vi "FileAppenderConfigDTOFromNative.vi"(8 "error in (no error)":errorcluster, 11 "FileAppenderConfig":T1={"common"={"id"="", "threshold"=enum."INFO", "filter"={"mode"=enum."Mirror", "levelMin"=enum."INFO", "levelMax"=enum."INFO", "tagPrefix"=""}, "queueBound"=0, "dropPolicy"=enum."DropOldest", "useUTC"=FALSE}, "file"={"rootFolder"=path "", "maxFileSize"=0, "maxFileCount"=0, "baseName"="", "extension"="", "delimiter"="", "calendarFolderTree"=FALSE}}) -> (0 "error out":errorcluster, 3 "FileAppenderConfigDTO":T8={"common"={"id"="", "threshold"="INFO", "filter"={"mode"="Mirror", "levelMin"="INFO", "levelMax"="INFO", "tagPrefix"=""}, "queueBound"=0, "dropPolicy"="DropOldest", "useUTC"=FALSE}, "file"={"rootFolder"="", "maxFileSize"=0, "maxFileCount"=0, "baseName"="", "extension"="", "delimiter"="", "calendarFolderTree"=FALSE}})   [LabVIEW 2026, in "Lumberjack.lvlib"]
uses:
  Lumberjack.lvlib
  TypeDefs/ConfigDTO/FilterDTO.ctl
  TypeDefs/ConfigDTO/AppenderConfigDTO.ctl
  TypeDefs/ConfigDTO/FileAppenderConfigDTO.ctl
  TypeDefs/ConfigDTO/FileConfigDTO.ctl
  TypeDefs/Severity.ctl
  TypeDefs/FilterMode.ctl
  TypeDefs/Filter.ctl
  TypeDefs/DropPolicy.ctl
  TypeDefs/AppenderConfig.ctl
  TypeDefs/FileAppenderConfig.ctl
  TypeDefs/FileConfig.ctl
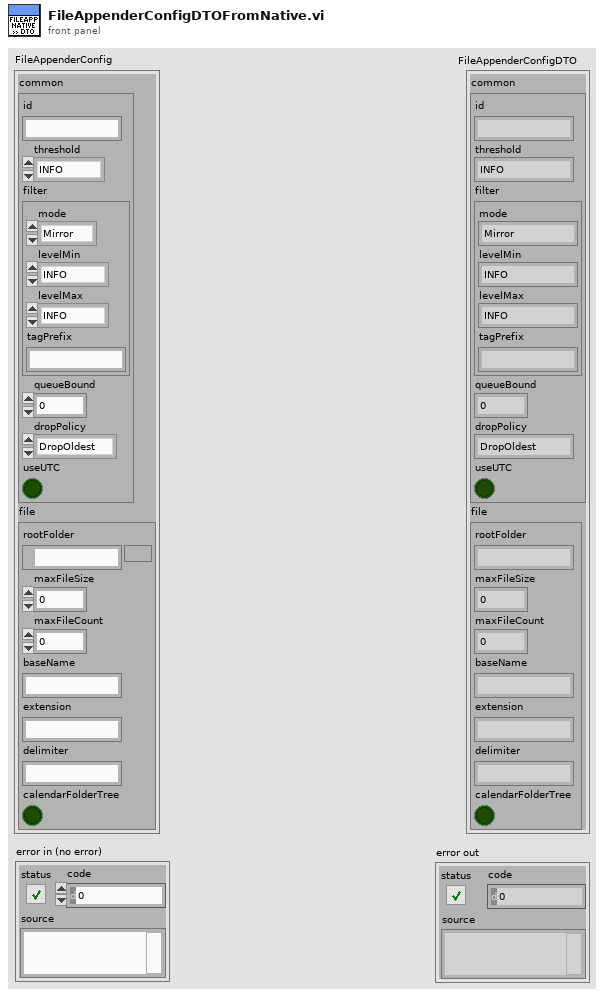
[diagram p1: front panel]
types:
  T1 = typedef "Lumberjack.lvlib/FileAppenderConfig.ctl" = cluster{"common":T2, "file":T7}
  T2 = typedef "Lumberjack.lvlib/AppenderConfig.ctl" = cluster{"id":string, "threshold":T3, "filter":T4, "queueBound":i32, "dropPolicy":T6, "useUTC":bool}
  T3 = typedef "Lumberjack.lvlib/Severity.ctl" = enum16{"OFF", "FATAL", "ERROR", "WARN", "INFO", "DEBUG", "TRACE", "ALL"}
  T4 = typedef "Lumberjack.lvlib/Filter.ctl" = cluster{"mode":T5, "levelMin":T3, "levelMax":T3, "tagPrefix":string}
  T5 = typedef "Lumberjack.lvlib/FilterMode.ctl" = enum16{"Mirror", "Routed"}
  T6 = typedef "Lumberjack.lvlib/DropPolicy.ctl" = enum16{"DropOldest", "DropNewest", "LevelAware"}
  T7 = typedef "Lumberjack.lvlib/FileConfig.ctl" = cluster{"rootFolder":path, "maxFileSize":i64, "maxFileCount":i32, "baseName":string, "extension":string, "delimiter":string, "calendarFolderTree":bool}
  T8 = typedef "Lumberjack.lvlib/FileAppenderConfigDTO.ctl" = cluster{"common":T9, "file":T11}
  T9 = typedef "Lumberjack.lvlib/AppenderConfigDTO.ctl" = cluster{"id":string, "threshold":string, "filter":T10, "queueBound":i32, "dropPolicy":string, "useUTC":bool}
  T10 = typedef "Lumberjack.lvlib/FilterDTO.ctl" = cluster{"mode":string, "levelMin":string, "levelMax":string, "tagPrefix":string}
  T11 = typedef "Lumberjack.lvlib/FileConfigDTO.ctl" = cluster{"rootFolder":string, "maxFileSize":i64, "maxFileCount":i32, "baseName":string, "extension":string, "delimiter":string, "calendarFolderTree":bool}
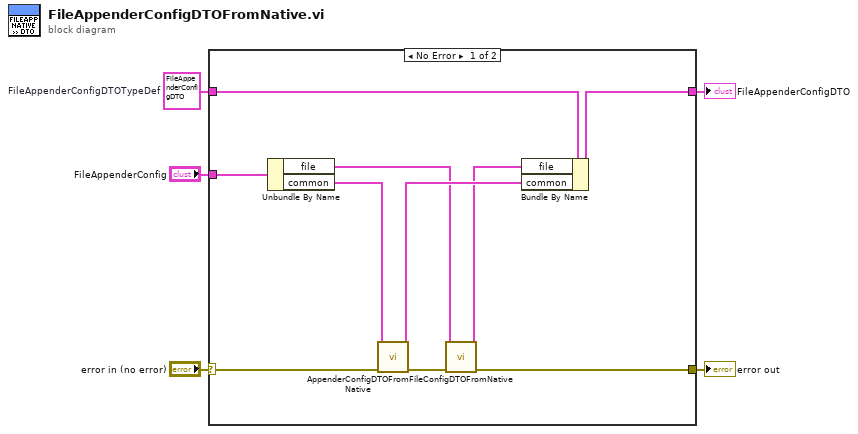
[diagram p0: block diagram]
diagram:
  w3 = T8 {"common"={"id"="", "threshold"="INFO", "filter"={"mode"="Mirror", "levelMin"="INFO", "levelMax"="INFO", "tagPrefix"=""}, "queueBound"=0, "dropPolicy"="DropOldest", "useUTC"=FALSE}, "file"={"rootFolder"="", "maxFileSize"=0, "maxFileCount"=0, "baseName"="", "extension"="", "delimiter"="", "calendarFolderTree"=FALSE}}  # FileAppenderConfigDTOTypeDef
  n1 = case shown="No Error" "error in (no error)" {
    selector: "error in (no error)" -> [w15 w17]
    tunnel: [w6 w17] -> w1
    tunnel: "FileAppenderConfig" -> [w13 _]
    tunnel: [w14 w16] -> w2
    tunnel: w3 -> [w12 w16]
    frame No Error {
      n2 = Unbundle By Name(w13) -> ("file"=w9:T7, "common"=w11:T2)
      n3 = call "AppenderConfigDTOFromNative.vi"("error in (no error)"=w15, "AppenderConfig"=w11) -> ("error out"=w7:errorcluster, "AppenderConfigDTO"=w10:T9)  [unwired: 8 in]
      n4 = call "FileConfigDTOFromNative.vi"("error in (no error)"=w7, "FileConfig"=w9) -> ("error out"=w6:errorcluster, "FileConfigDTO"=w8:T11)  [unwired: 8 in]
      n5 = Bundle By Name(cluster=w12, "file"=w8, "common"=w10) -> (w14:T8)
    }
    frame Error {
    }
  }
  "error out" <- w1
  "FileAppenderConfigDTO" <- w2
